vi "BlkXfer.vi"(0 "VISA IN":refnum<visa-resource-name>="GPIB1::16::INSTR", 1 "FileName":string, 5 "error in":errorcluster, 7 "Channel":i32=1) -> (14 "VISA Out":refnum<visa-resource-name>="GPIB1::16::INSTR", 16 "Data":dbl[](array[numeric]), 19 "error out":errorcluster={"status"=TRUE, "code"=-1074001424, "source"="BlkXfer.vi -> Instrument Error: 106: +106,\"Requested measurement not found\""})   [LabVIEW 2018, in "PNA-X.lvlib"]
uses:
  PNA-X.lvlib
panel:
  out "Waveform Chart":dbl[](graph)
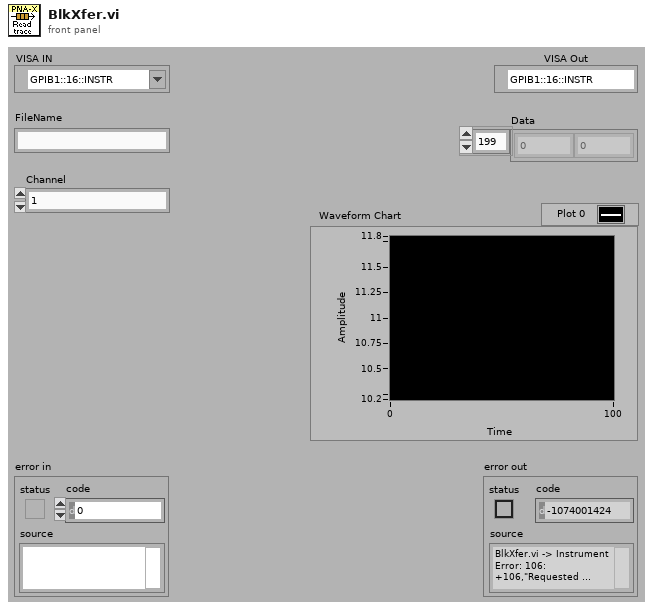
[diagram p1: front panel]
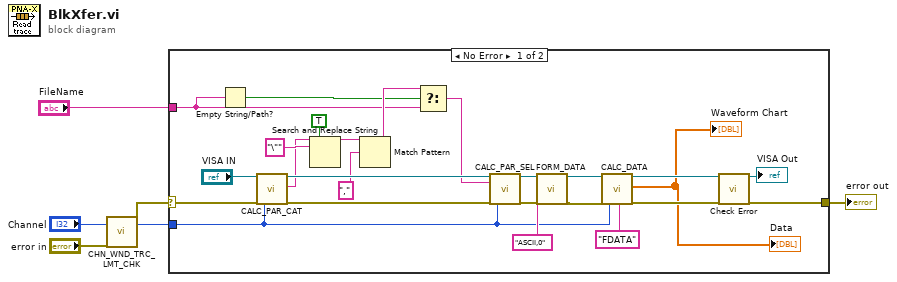
[diagram p0: block diagram]
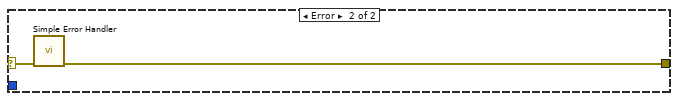
[diagram p2: hidden frame]
diagram:
  n1 = call "CHN_WND_TRC_LMT_CHK.vi"("Channel"="Channel", "error in"="error in") -> ("error out"=w4:errorcluster, "Channel"=w3:i32)  [unwired: 13 in, 3 out]
  n2 = case shown="No Error" w4 {
    selector: w4 -> [w27 w33]
    tunnel: [w31 w32] -> w5
    tunnel: w3 -> [w15 _]
    tunnel: "FileName" -> [w8 _]
    frame No Error {
      n3 = Empty String/Path?(string/path=w8) -> (empty?=w9:bool)
      n4 = call "CALC_PAR_CAT.vi"("VISA IN"="VISA IN", "error in"=w27, "Channel"=w15) -> ("VISA Out"=w29:refnum<visa-resource-name>, "Data"=w21:string, "error out"=w26:errorcluster)  [unwired: 12 in, 2 out]
      n5 = Search and Replace String(replace all?=TRUE ("replace all? (F)"), input string=w21, search string="\"") -> (result string=w24:string)  [unwired: 5 in, 3 out]
      n6 = Match Pattern(string=w24, regular expression=",") -> (before substring=w10:string)  [unwired: 1 in, 3 out]
      n7 = Select(t=w10, s=w9, f=w8) -> (s? t:f=w7:string)
      n8 = call "CALC_PAR_SEL.vi"("VISA IN"=w29, "Measurement"=w7, "error in"=w26, "Channel"=w15) -> ("VISA Out"=w20:refnum<visa-resource-name>, "error out"=w19:errorcluster)  [unwired: 14 in]
      n9 = call "FORM_DATA.vi"("VISA IN"=w20, "error in"=w19, "DataType"="ASCII,0") -> ("VISA Out"=w16:refnum<visa-resource-name>, "error out"=w17:errorcluster)  [unwired: 15 in]
      n10 = call "CALC_DATA.vi"("VISA IN"=w16, "error in"=w17, "Channel"=w15, "DataType"="FDATA") -> ("VISA Out"=w12:refnum<visa-resource-name>, "array"=→"Data" →"Waveform Chart":dbl[], "error out"=w13:errorcluster)  [unwired: 13 in]
      n11 = call "Check Error.vi"("VISA Resource Name"=w12, "error in (no error)"=w13) -> ("dup VISA session"=→"VISA Out":refnum<visa-resource-name>, "error out"=w31:errorcluster)  [unwired: 16 in]
    }
    frame Error {
      n12 = call <vilib>:"Simple Error Handler.vi"("error in (no error)"=w33) -> ("error out"=w32:errorcluster)  [unwired: 4 in, 4 out]
    }
  }
  "error out" <- w5
